vi "Helper SubVI - Mode Parameter.vi"(6 "mode index":i32, 8 "phase":dbl[][](array[numeric]), 9 "mag":dbl[][](array[numeric]), 10 "damping in":dbl[](array[numeric]), 11 "freq in":dbl[](array[numeric])) -> (1 "mode shape":dbl[][](array[numeric]), 2 "damping out":dbl[](array[numeric]), 3 "freq out":dbl[](array[numeric]))   [LabVIEW 2023]
doc: "Obtains the natural frequency, damping ratio, and modal shape for each mode of the aluminum plate."
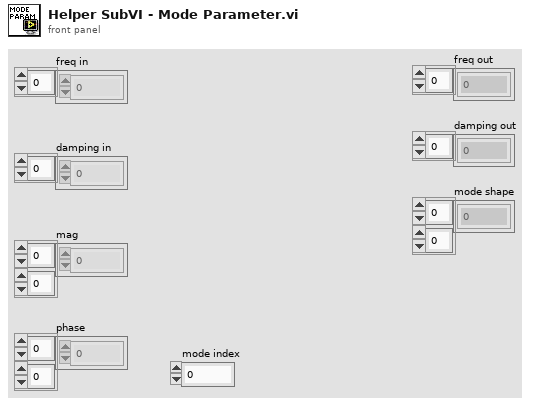
[diagram p1: front panel]
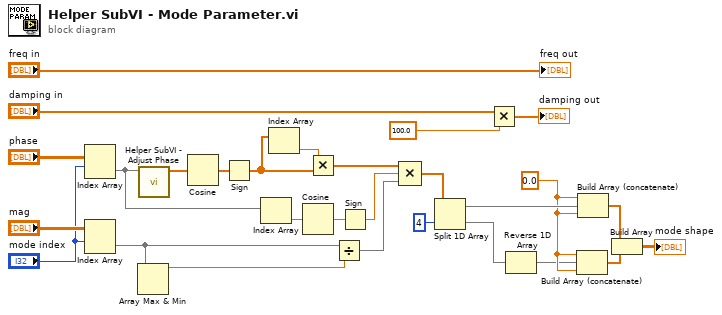
[diagram p0: block diagram]
diagram:
  w7 = 0.0 ("disabled index (col)")
  n1 = Index Array(array="phase", index (row)="mode index") -> (element=w2:dbl[])  [unwired: 1 in]
  n2 = Index Array(array="mag", index (row)="mode index") -> (element=w27:dbl[])  [unwired: 1 in]
  n3 = Array Max & Min(array=w27) -> (max value=w28:dbl)  [unwired: 3 out]
  n4 = call "Helper SubVI - Adjust Phase.vi"("Phase"=w2) -> ("Adjusted phase"=w1:dbl[])  [unwired: 10 in]
  n5 = Cosine(x=w1) -> (cos(x)=w15:dbl[])
  n6 = Sign(1:w15) -> (0:w13:dbl[])
  n7 = Index Array(array=w2) -> (element=w16:dbl)  [unwired: 1 in]
  n8 = Index Array(array=w13) -> (element=w14:dbl)  [unwired: 1 in]
  n9 = Cosine(x=w16) -> (cos(x)=w18:dbl)
  n10 = Multiply(x=w14, y=w13) -> (x*y=w12:dbl[])
  n11 = Divide(x=w27, y=w28) -> (x/y=w19:dbl[])
  n12 = Sign(1:w18) -> (0:w17:dbl)
  n13 = Compound Arithmetic op=MULTIPLY(w12, w17, w19) -> (w10:dbl[])
  n14 = Split 1D Array(array=w10, index=4) -> (first subarray=w9:dbl[], second subarray=w8:dbl[])
  n15 = Multiply(x="damping in", y=100.0 ("disabled index (col)")) -> (x*y=→"damping out":dbl[])
  n16 = Reverse 1D Array(array=w8) -> (reversed array=w3:dbl[])
  n17 = Build Array (concatenate)(w7, w3, w7) -> (w6:dbl[])
  n18 = Build Array (concatenate)(w7, w9, w7) -> (w5:dbl[])
  n19 = Build Array(w5, w6) -> (→"mode shape":dbl[][])
  "freq out" <- "freq in"
